vi "SelectMenu3.vi"(6 "Click Type":T1, 7 "Id":string, 8 "Point":T3, 9 "Item Index":u32, 10 "XRef":refnum<vi>, 11 "State In":T2) -> (0 "Reply":string[](array[string]), 3 "State Out":T2)   [LabVIEW 2012, in "CThread.lvlib" / "CThread VI Terminal Node.xnode"]
doc: "This ability VI is called after the user selects an item from a portion of the menu defined during BuildMenu. Click Type is the type of click that led to the building of the menu whose selection is being handled by this VI. ItemIndex is the index of the element in the array used when you specified the popup menu. Id is the id you associated with the item in BuildMenu3. Point is the location where the user clicked to build the menu relative to the top-left corner of the XNode. You can display a dialog in response to a user selection if you wish. Use Reply to inform LabVIEW of any actions it needs to take.\n\nDefault behavior: None.\n\nThis ability provides UI and OS messages are handled.\n\nSee also: BuildMenu3"
uses:
  CThread VI Terminal Node.xnode
  State.ctl
  <vilib>/XNodeSupport/XNodePoint.ctl
  <vilib>/XNodeSupport/XNodeInt.ctl
  <vilib>/XNodeSupport/XNodeClickTypes.ctl
  <vilib>/_script/New VI Object TypeDefs/NewVIObject_LVRelativePositionTypeDef.ctl
  <vilib>/_script/New VI Object TypeDefs/NewVIObject_LVRelativeDirectionTypeDef.ctl
  <vilib>/Utility/miscctls.llb/LVPoint32TypeDef.ctl
  referencenode/Image.vi
  referencenode/CThread VI Reference.xnode
  CThread.lvlib
  <vilib>/XNodeSupport/NI_XNodeSupport.lvlib
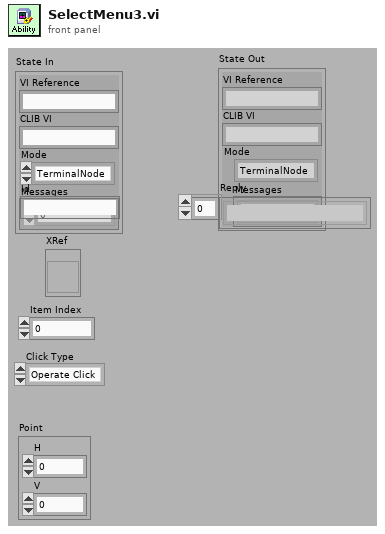
[diagram p1: front panel]
types:
  T1 = typedef "NI_XNodeSupport.lvlib/XNodeClickTypes.ctl" = enum32{"Operate Click", "Popup Click"}
  T2 = typedef "CThread.lvlib/CThread VI Terminal Node.xnode/State.ctl" = cluster{"VI Reference":string, "CLIB VI":string, "Mode":enum16{"TerminalNode", "AdaptorNode"}, "Messages":u8[]}
  T3 = typedef "NI_XNodeSupport.lvlib/XNodePoint.ctl" = cluster{"H":T4, "V":T4}
  T4 = typedef "NI_XNodeSupport.lvlib/XNodeInt.ctl" = i32
  T5 = typedef "NewVIObject_LVRelativePositionTypeDef.ctl" = cluster{"Refnum":refnum<vi>, "Relative Direction":T6, "Point32":T7}
  T6 = typedef "NewVIObject_LVRelativeDirectionTypeDef.ctl" = enum32{"Right", "Left", "Top", "Bottom", "Top Right", "Top Left", "Bottom Right", "Bottom Left"}
  T7 = typedef "LVPoint32TypeDef.ctl" = cluster{"Horizontal":i32, "Vertical":i32}
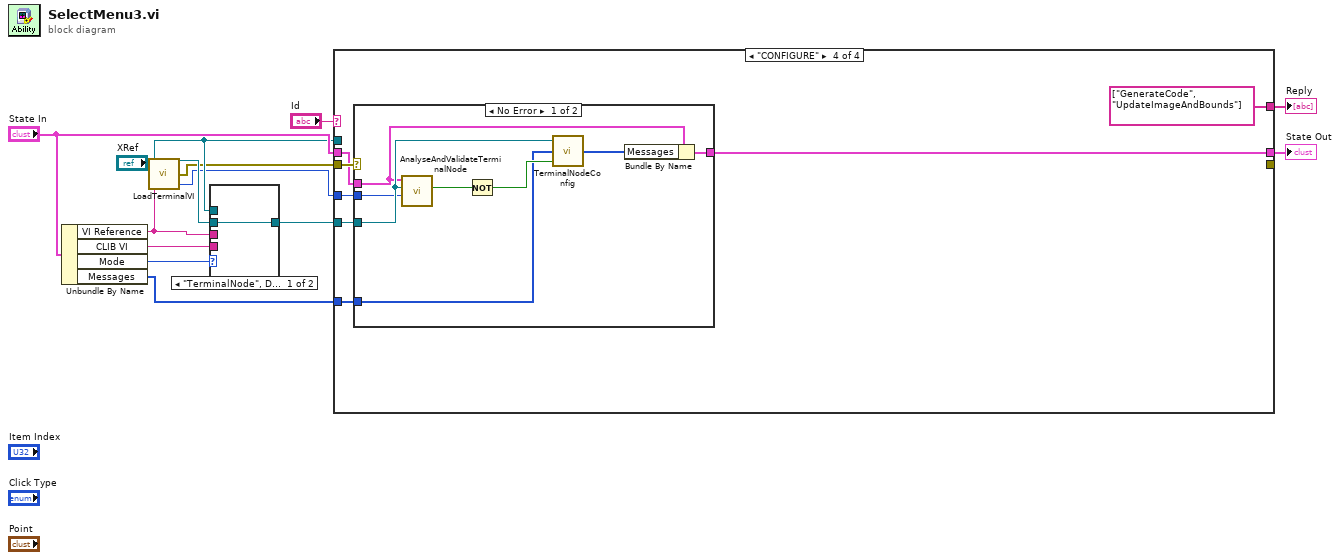
[diagram p0: block diagram]
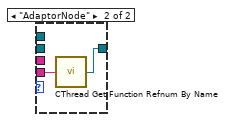
[diagram p2: hidden frame]
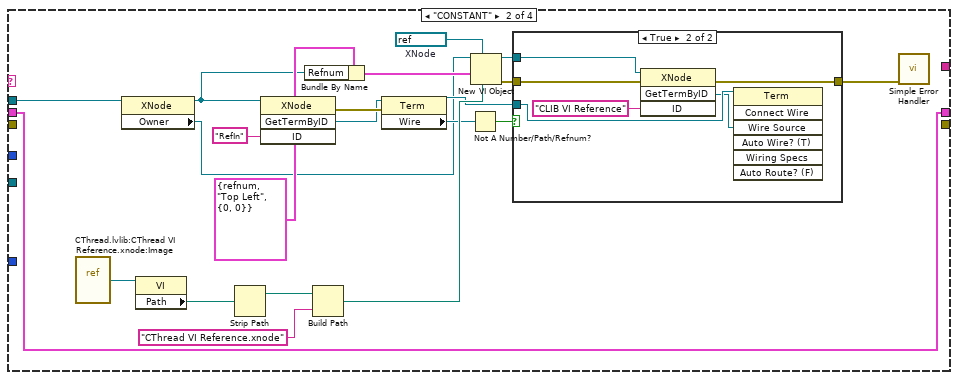
[diagram p4: hidden frame]
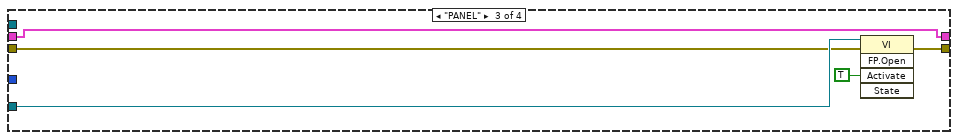
[diagram p6: hidden frame]
diagram:
  n1 = Unbundle By Name("State In") -> ("VI Reference"=w4:string, "CLIB VI"=w10:string, "Mode"=w11:enum16{"TerminalNode", "AdaptorNode"}, "Messages"=w6:u8[])
  n2 = call "LoadTerminalVI.vi"("VI Reference"=w4, "XRef"="XRef") -> ("Clone Number"=w1:i16, "error out"=w2:errorcluster, "vi reference"=w3:refnum<vi>)  [unwired: 1 in]
  n3 = case shown="\"TerminalNode\", Default" w11 {
    tunnel: w4 -> [_ _]
    tunnel: w10 -> [_ w16]
    tunnel: [w14 w15] -> w8
    tunnel: "XRef" -> [_ _]
    tunnel: w3 -> [w14 _]
    frame "TerminalNode", Default {
    }
    frame "AdaptorNode" {
      n4 = call "CThread Get Function Refnum By Name.vi"("Name"=w16) -> ("vi reference"=w15:refnum<vi>)  [unwired: 2 out]
    }
  }
  n5 = case shown="\"CONFIGURE\"" "Id" {
    tunnel: "XRef" -> [_ w37 _ _]
    tunnel: [_ _ _ string[] ["GenerateCode", "UpdateImageAndBounds"] ("Reply")] -> w12
    tunnel: [_ _ w49 _] -> _
    tunnel: "State In" -> [w17 w18 w46 w54]
    tunnel: w8 -> [_ _ w48 w56]
    tunnel: w2 -> [_ _ w47 w55]
    tunnel: [w17 w18 w46 w53] -> w7
    tunnel: w6 -> [_ _ _ w52]
    tunnel: w1 -> [_ _ _ w51]
    frame Default {
    }
    frame "CONSTANT" {
      w36 = refnum<vi> refnum  # XNode
      n6 = vi-ref "CThread.lvlib:CThread VI Reference.xnode:Image.vi"() -> (w21:refnum<vi>)
      n7 = property class="XNode"(reference=w37) -> (reference out=w26:refnum<vi>, "Owner"=w24:refnum<vi>)  [unwired: 1 in, 1 out]
      n8 = property class="VI"(reference=w21) -> ("Path"=w20:path)  [unwired: 1 in, 2 out]
      n9 = Strip Path(path=w20) -> (stripped path=w19:path)  [unwired: 1 out]
      n10 = invoke class="XNode" method="GetTermByID"(reference=w26, "ID"="RefIn") -> (error out=w32:errorcluster, "GetTermByID"=w31:refnum<vi>)  [unwired: 2 in, 2 out]
      n11 = Bundle By Name(cluster=T5 {"Refnum"=refnum, "Relative Direction"=enum."Top Left", "Point32"={"Horizontal"=0, "Vertical"=0}} ("Relative Position"), "Refnum"=w26) -> (w25:T5)
      n12 = Build Path(base path=w19, name or relative path="CThread VI Reference.xnode") -> (appended path=w35:path)
      n13 = property class="Term"(reference=w31, error in=w32) -> (reference out=w28:refnum<vi>, "Wire"=w30:refnum<vi>)  [unwired: 1 out]
      n14 = Not A Number/Path/Refnum?(number/path/refnum=w30) -> (NaN/Path/Refnum?=w29:bool)
      n15 = New VI Object(vi object class=w36, owner refnum=w24, position/next to=w25, 6:w35) -> (object refnum=w22:refnum<vi>, 0:w23:errorcluster)  [unwired: 4 in]
      n16 = case shown="True" w29 {
        tunnel: w28 -> [_ w43]
        tunnel: [w39 w40] -> w34
        tunnel: w22 -> [_ w45]
        tunnel: w23 -> [w39 w44]
        frame False {
        }
        frame True {
          n17 = invoke class="XNode" method="GetTermByID"(reference=w45, error in=w44, "ID"="CLIB VI Reference") -> (error out=w40:errorcluster, "GetTermByID"=w42:refnum<vi>)  [unwired: 1 in, 2 out]
          n18 = invoke class="Term" method="Connect Wire"(reference=w43, "Wire Source"=w42) -> ()  [unwired: 5 in, 7 out]
        }
      }
      n19 = call <vilib>:"Simple Error Handler.vi"("error in (no error)"=w34) -> ()  [unwired: 4 in, 5 out]
    }
    frame "PANEL" {
      n20 = invoke class="VI" method="FP.Open"(reference=w48, error in=w47, "Activate"=TRUE ("Activate?")) -> (error out=w49:errorcluster)  [unwired: 2 in, 4 out]
    }
    frame "CONFIGURE" {
      n21 = case shown="No Error" w55 {
        tunnel: w56 -> [w62 _]
        tunnel: w54 -> [w61 w66]
        tunnel: [w60 w66] -> w53
        tunnel: w52 -> [w59 _]
        tunnel: w51 -> [w58 _]
        frame No Error {
          n22 = call "AnalyseAndValidateTerminalNode.vi"("CloneID"=w58, "Comparison VI"=w62, "State"=w61) -> ("Valid"=w64:bool)  [unwired: 5 in, 3 out]
          n23 = Not(x=w64) -> (.not. x?=w65:bool)
          n24 = call "TerminalNodeConfig.vi"("reference"=w62, "Old Messages"=w59, "Reconf?"=w65) -> ("Messages"=w63:u8[])  [unwired: 6 in]
          n25 = Bundle By Name(cluster=w61, "Messages"=w63) -> (w60:T2)
        }
        frame Error {
        }
      }
    }
  }
  "State Out" <- w7
  "Reply" <- w12
